vi "Login.vi"(7 "LabVIEW Web Service Request":refnum<class "Web Request.lvclass">) -> ()   [LabVIEW 2014]
uses:
  <vilib>/wsapi/Web Request.lvclass
  <vilib>/wsapi/class/subVIs/Write Single Session Variable.vi
  Coding Platform.lvlib
panel:
  # "Use the Web Service Request input terminal to call the VIs on the Web Services palette. Do not remove it from the connector pane unless you don't need access to the palette."
  # "Each additional control wired to the connector pane will be available as an input in the URL. To include an indicator in terminal-mode output (the default setting), it must also be wired to the connector pane."
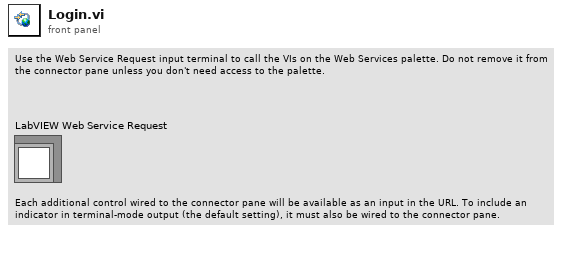
[diagram p1: front panel]
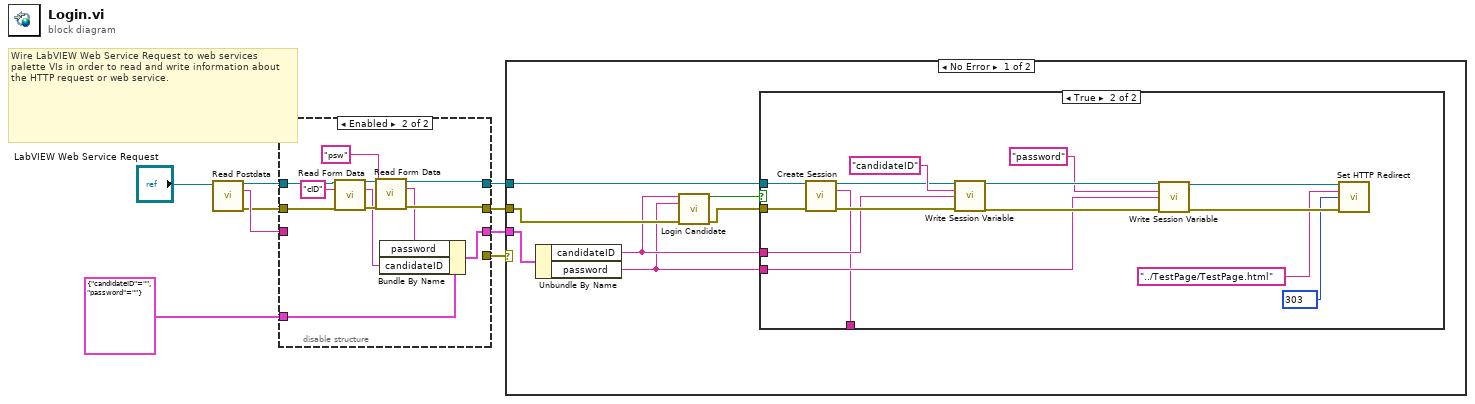
[diagram p0: block diagram]
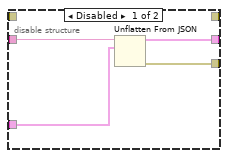
[diagram p2: hidden frame]
diagram:
  # "Wire LabVIEW Web Service Request to web services palette VIs in order to read and write information about the HTTP request or web service."
  n1 = call <vilib>:"Read Postdata.vi"("LabVIEW Web Service Request"="LabVIEW Web Service Request") -> ("LabVIEW Web Service Request out"=w3:refnum<class "Web Request.lvclass">, "postdata"=w8:string, "error out"=w1:errorcluster)  [unwired: 12 in]
  n2 = disable-structure shown="Enabled" {
    disable-tunnel: w8 -> [w13 _]
    disable-tunnel: cluster{"candidateID":string, "password":string} {"candidateID"="", "password"=""} -> [w12 w18]
    disable-tunnel: [w11 _] -> w6
    disable-tunnel: [w10 w17] -> w5
    disable-tunnel: [_ w23] -> w4
    disable-tunnel: w3 -> [_ w25]
    disable-tunnel: [_ w20] -> w2
    disable-tunnel: w1 -> [_ w22]
    frame Disabled {
      n3 = Unflatten From JSON(JSON string=w13, type and defaults=w12) -> (value=w10:cluster{"candidateID":string, "password":string}, error out=w11:errorcluster)  [unwired: 5 in]
    }
    frame Enabled {
      n4 = call <vilib>:"Read Form Data.vi"("LabVIEW Web Service Request"=w25, "key"="cID", "error in (no error)"=w22) -> ("LabVIEW Web Service Request out"=w24:refnum<class "Web Request.lvclass">, "value"=w14:string, "error out"=w21:errorcluster)  [unwired: 9 in, 1 out]
      n5 = call <vilib>:"Read Form Data.vi"("LabVIEW Web Service Request"=w24, "key"="psw", "error in (no error)"=w21) -> ("LabVIEW Web Service Request out"=w23:refnum<class "Web Request.lvclass">, "value"=w15:string, "error out"=w20:errorcluster)  [unwired: 9 in, 1 out]
      n6 = Bundle By Name(cluster=w18, "password"=w15, "candidateID"=w14) -> (w17:cluster{"candidateID":string, "password":string})
    }
  }
  n7 = case shown="No Error" w6 {
    tunnel: w4 -> [w32 _]
    tunnel: w5 -> [w31 _]
    tunnel: w2 -> [w30 _]
    frame No Error {
      n8 = Unbundle By Name(w31) -> ("candidateID"=w27:string, "password"=w26:string)
      n9 = call "Login Candidate.vi"("Candidate ID"=w27, "Password"=w26, "error in (no error)"=w30) -> ("LoggedIn"=w28:bool, "error out"=w29:errorcluster)  [unwired: 11 in]
      n10 = case shown="True" w28 {
        tunnel: w32 -> [_ w45]
        tunnel: w29 -> [_ w44]
        tunnel: w27 -> [_ w37]
        tunnel: w26 -> [_ w36]
        tunnel: [_ w33] -> _
        frame False {
        }
        frame True {
          w34 = 303 items=["100"=100, "101"=101, "200"=200, "201"=201, "202"=202, "203"=203, "204"=204, "205"=205, "206"=206, "300"=300, "301"=301, "302"=302, "303"=303, "304"=304, "305"=305, "306"=306, "307"=307, "400"=400, "401"=401, "402"=402, "403"=403, "404"=404, "405"=405, "406"=406, "407"=407, "408"=408, "409"=409, "410"=410, "411"=411, "412"=412, "413"=413, "414"=414, "415"=415, "416"=416, "417"=417, "500"=500, "501"=501, "502"=502, "503"=503, "504"=504, "505"=505] ("response code (307)")
          n11 = call <vilib>:"Create Session.vi"("LabVIEW Web Service Request"=w45) -> ("LabVIEW Web Service Request out"=w35:refnum<class "Web Request.lvclass">, "session ID cookie"=w33:string)  [unwired: 12 in, 1 out]
          n12 = call-poly <vilib>:"Write Session Variable.vi"("LabVIEW Web Service Request"=w35, "key"="candidateID", "value"=w37, "error in (no error)"=w44) -> ("LabVIEW Web Service Request out"=w43:refnum<class "Web Request.lvclass">, "error out"=w40:errorcluster)  [unwired: 8 in, 2 out]
          n13 = call-poly <vilib>:"Write Session Variable.vi"("LabVIEW Web Service Request"=w43, "key"="password", "value"=w36, "error in (no error)"=w40) -> ("LabVIEW Web Service Request out"=w39:refnum<class "Web Request.lvclass">, "error out"=w41:errorcluster)  [unwired: 8 in, 2 out]
          n14 = call <vilib>:"Set HTTP Redirect.vi"("LabVIEW Web Service Request"=w39, "redirect URL"="../TestPage/TestPage.html", "response code (307)"=w34, "error in (no error)"=w41) -> ()  [unwired: 10 in, 2 out]
        }
      }
    }
    frame Error {
    }
  }
